vi "DI IRQ GetErrors.vi"(0 "XRef":T14, 1 "Generate Strings?":T2, 2 "State In":T6) -> (14 "Errors":T3, 15 "Errors Present?":T2, 16 "Fatal Error Out":T1)   [LabVIEW 2021, in "myRIO Register DI IRQ.xnode"]
uses:
  <vilib>/myRIO/Instrument Drivers/IRQ/IO IRQ/vis/myRIO Register DI IRQ.xnode
  <vilib>/XNodeSupport/XNodeXNodeRef.ctl
  <vilib>/XNodeSupport/XNodeBool.ctl
  <vilib>/myRIO/Instrument Drivers/IRQ/IO IRQ/vis/DI IRQ State.ctl
  <vilib>/myRIO/Common/Instrument Driver Framework/Utilities/typedefs/myRIOXPeripheral.ctl
  <vilib>/XNodeSupport/XNodeTerm4Array.ctl
  <vilib>/XNodeSupport/XNodeTerm4.ctl
  <vilib>/XNodeSupport/XNodeString.ctl
  <vilib>/XNodeSupport/XNodeVariant.ctl
  <vilib>/XNodeSupport/XNodeRect32.ctl
  <vilib>/XNodeSupport/XNodeInt.ctl
  <vilib>/XNodeSupport/XNodeTermDirection.ctl
  <vilib>/XNodeSupport/XNodeError3Array.ctl
  <vilib>/XNodeSupport/XNodeError3.ctl
  <vilib>/XNodeSupport/XNodeErrorCluster.ctl
  <vilib>/XNodeSupport/NI_XNodeSupport.lvlib
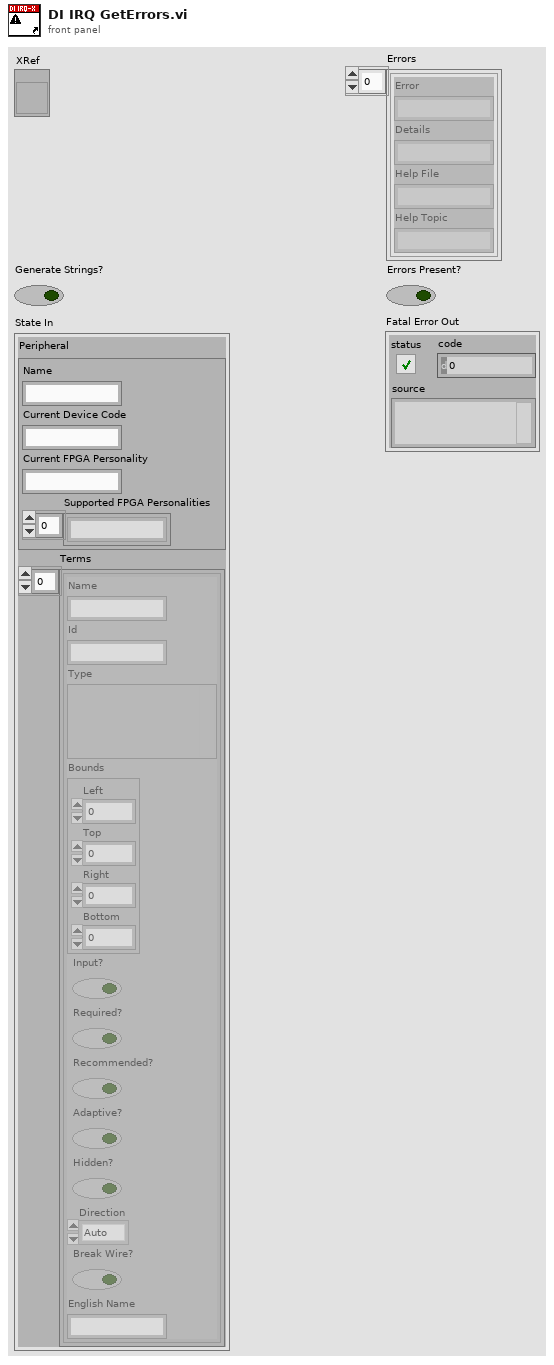
[diagram p1: front panel]
types:
  T1 = typedef "NI_XNodeSupport.lvlib/XNodeErrorCluster.ctl" = errorcluster
  T2 = typedef "NI_XNodeSupport.lvlib/XNodeBool.ctl" = bool
  T3 = typedef "NI_XNodeSupport.lvlib/XNodeError3Array.ctl" = T4[]
  T4 = typedef "NI_XNodeSupport.lvlib/XNodeError3.ctl" = cluster{"Error":T5, "Details":T5, "Help File":T5, "Help Topic":T5}
  T5 = typedef "NI_XNodeSupport.lvlib/XNodeString.ctl" = string
  T6 = typedef "myRIO Register DI IRQ.xnode/DI IRQ State.ctl" = cluster{"Peripheral":T7, "Terms":T8}
  T7 = typedef "myRIOXPeripheral.ctl" = cluster{"Name":string, "Current Device Code":string, "Current FPGA Personality":string, "Supported FPGA Personalities":string[]}
  T8 = typedef "NI_XNodeSupport.lvlib/XNodeTerm4Array.ctl" = T9[]
  T9 = typedef "NI_XNodeSupport.lvlib/XNodeTerm4.ctl" = cluster{"Name":T5, "Id":T5, "Type":T10, "Bounds":T11, "Input?":T2, "Required?":T2, "Recommended?":T2, "Adaptive?":T2, "Hidden?":T2, "Direction":T13, "Break Wire?":T2, "English Name":T5}
  T10 = typedef "NI_XNodeSupport.lvlib/XNodeVariant.ctl" = variant
  T11 = typedef "NI_XNodeSupport.lvlib/XNodeRect32.ctl" = cluster{"Left":T12, "Top":T12, "Right":T12, "Bottom":T12}
  T12 = typedef "NI_XNodeSupport.lvlib/XNodeInt.ctl" = i32
  T13 = typedef "NI_XNodeSupport.lvlib/XNodeTermDirection.ctl" = enum32{"Auto", "Up", "Down", "Left", "Right", "Center"}
  T14 = typedef "NI_XNodeSupport.lvlib/XNodeXNodeRef.ctl" = refnum<vi>
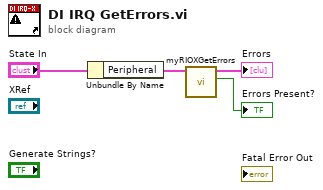
[diagram p0: block diagram]
diagram:
  n1 = Unbundle By Name("State In") -> ("Peripheral"=w1:T7)
  n2 = call <vilib>:"myRIOXGetErrors.vi"("Peripheral"=w1) -> ("Errors Present?"=→"Errors Present?":T2, "Errors"=→"Errors":T4[])  [unwired: 9 in]
